vi "ev Panel close.vi"(8 "error in (no error)":errorcluster, 11 "LF2R IDE in":refnum<class "LF2R IDE.lvclass">) -> (0 "error out":errorcluster, 3 "LF2R IDE out":refnum<class "LF2R IDE.lvclass">)   [LabVIEW 2018, in "LF2R IDE.lvlib" / "LF2R IDE.lvclass"]
uses:
  LF2R IDE.lvclass
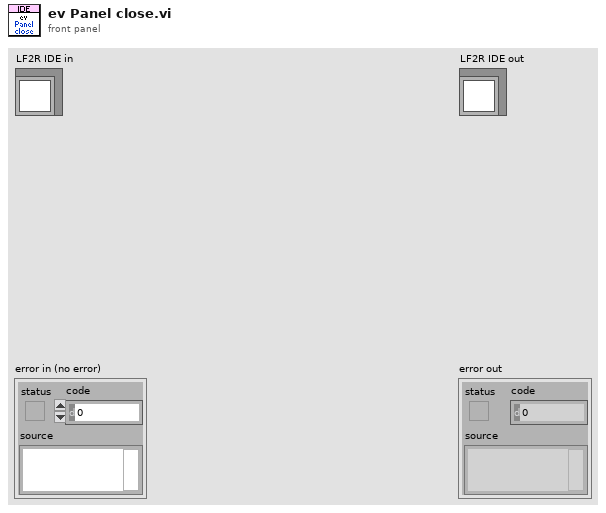
[diagram p1: front panel]
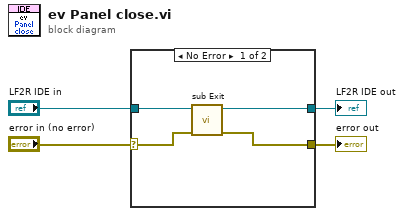
[diagram p0: block diagram]
diagram:
  n1 = case shown="No Error" "error in (no error)" {
    selector: "error in (no error)" -> [w6 w10]
    tunnel: [w5 w10] -> w3
    tunnel: [w7 w9] -> w1
    tunnel: "LF2R IDE in" -> [w8 w9]
    frame No Error {
      n2 = call "sub Exit.vi"("error in (no error)"=w6, "LF2R IDE in"=w8) -> ("error out"=w5:errorcluster, "LF2R IDE out"=w7:refnum<class "LF2R IDE.lvclass">)  [unwired: 8 in]
    }
    frame Error {
    }
  }
  "error out" <- w3
  "LF2R IDE out" <- w1
